vi "DAQ.44xx.Get Dev Product Type.vi"(8 "error in (no error)":errorcluster, 11 "Refnum in":refnum<k21>) -> (0 "error out":errorcluster, 1 "DevIsSimulated":bool, 2 "DAQ Type":T1, 3 "Refnum out":refnum<k21>)   [LabVIEW 2019, in "Instrument.DAQ.lvclass"]
uses:
  Instrument.DAQ.lvclass
  Typedefs/DAQ.Type--enum.ctl
  <resource>/objmgr/daqmx.rc
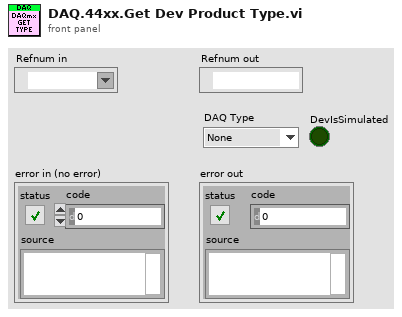
[diagram p1: front panel]
types:
  T1 = typedef "Instrument.DAQ.lvclass/DAQ.Type--enum.ctl" = enum16{"None", "USB 4431", "PXI 446x"}
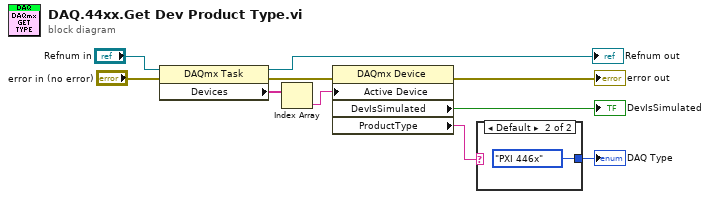
[diagram p0: block diagram]
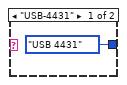
[diagram p2: hidden frame]
diagram:
  n1 = property class="DAQmx Task"(reference="Refnum in", error in="error in (no error)") -> (reference out=→"Refnum out":refnum<k21>, error out=w9:errorcluster, "Devices"=w1:tag[])
  n2 = Index Array(array=w1) -> (element=w3:tag)  [unwired: 1 in]
  n3 = property class="DAQmx Device"(error in=w9, "Active Device"=w3) -> (error out=→"error out":errorcluster, "DevIsSimulated"=→"DevIsSimulated":bool, "ProductType"=w2:string)  [unwired: 1 in, 1 out]
  n4 = case shown="Default" w2 {
    tunnel: [DAQ.Type--enum."USB 4431" ("DAQ Type") DAQ.Type--enum."PXI 446x" ("DAQ Type")] -> w5
    frame "USB-4431" {
    }
    frame Default {
    }
  }
  "DAQ Type" <- w5
